vi "Calibrate DataQ.vi"() -> ()   [LabVIEW 2024]
doc: "This example performs writes and reads on a serial port, as directed by the user. You can press the Write and Read buttons, and change the Read Count, while the example is running.\n\nThe parameters set for the serial port must match the parameters of the connected instrument or device. In this example, the Read Count parameter specifies the number of bytes that the serial port reads. If there were more bytes at the port than the specified number, those bytes would not be read. If there were less bytes at the port than the specified number, you would receive a timeout error.\n\nThis example expands upon the flow control options for XON and XOFF, allowing the user to choose those control characters. Also, the user can enable or disable a termination character. Some devices require a termination character in order to identify the end of command strings. Some devices send a termination character to signify the end of data to be read. This example shows how you can end the Read operation once a termination character is detected in the buffer and/or append a termination character at the end of the Write data."
uses:
  <vilib>/Instr/_visa.llb/VISA Configure Serial Port (Instr).vi
panel:
  out "read buffer":string
  out "size(s)":i32
  in  "Correction":dbl(slide) scale=-10.0..10.0
  in  "index (row)":i32
  in  "Cal Array":dbl[][](array[numeric])
  out "Scaled":dbl
  out "Measured IN":dbl
  out "Waveform Chart":dbl[](graph)
  in  "Command List":string="stop\nencode 0\nslist 0 0\nsrate 6000\nps 2\ndec 1\ndeca 3\nnop\n\n\n"
  in  "Stop":bool
  in  "2108 CDC Virtual COM":refnum<visa-resource-name>="COM3"
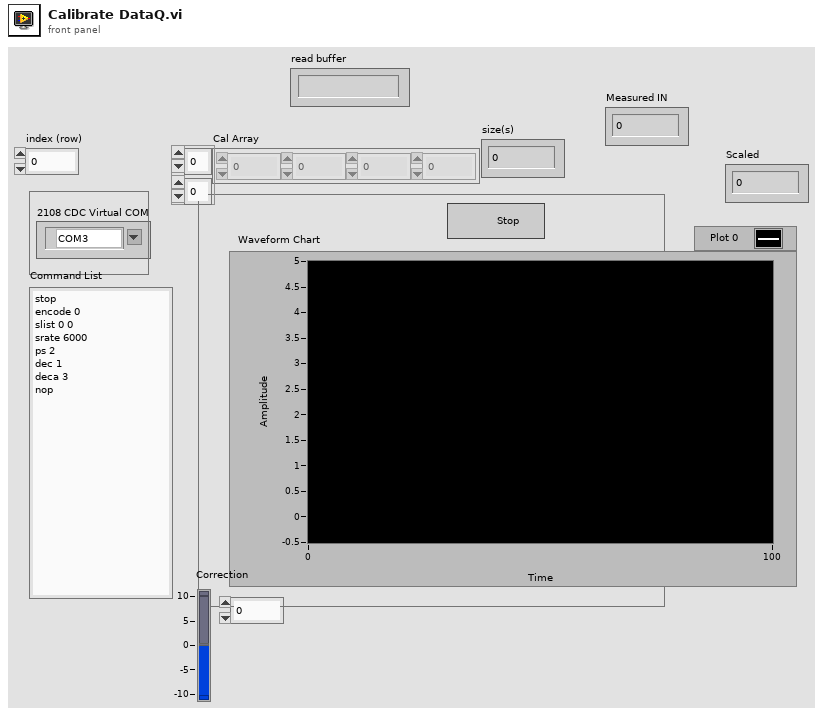
[diagram p1: front panel]
types:
  T1 = enum16{"big-endian, network order", "native, host order", "little-endian"}
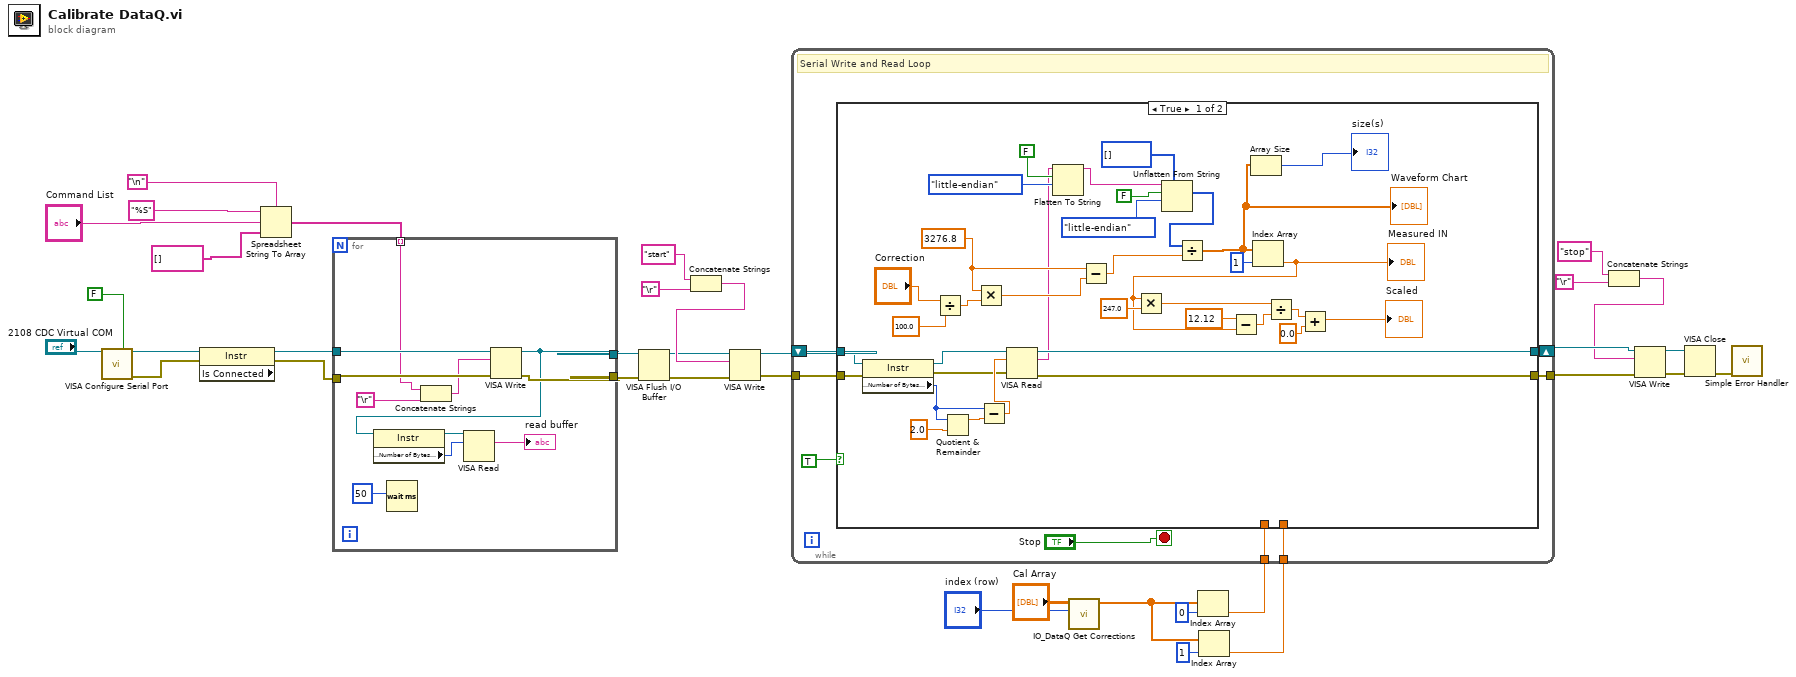
[diagram p0: block diagram]
diagram:
  n1 = call-poly "VISA Configure Serial Port"("VISA resource name"="2108 CDC Virtual COM", "Enable Termination\nChar (T)"=FALSE) -> ("VISA resource name out"=w33:refnum<visa-resource-name>, "error out"=w35:errorcluster)  [unwired: 8 in, 4 out]
  n2 = property class="Instr" props=["Is Connected"](reference=w33, error in=w35) -> (reference out=w9:refnum<visa-resource-name>, error out=w8:errorcluster)  [unwired: 1 out]
  n3 = Spreadsheet String To Array(delimiter (Tab)="\n", format string="%S", spreadsheet string="Command List", array type (2D Dbl)=string[] []) -> (array=w29:string[])
  n4 = for {
    tunnel: w29 -> [w43] mode=indexing
    tunnel: w9 -> [w46]
    tunnel: w8 -> [w45]
    tunnel: [w39] -> w13
    tunnel: [w40] -> w11
    n5 = Wait (ms)(milliseconds to wait=u32 50) -> ()  [unwired: 1 out]
    n6 = Concatenate Strings(w43, "\r") -> (w41:string)
    n7 = VISA Write(VISA resource name=w46, write buffer=w41, error in (no error)=w45) -> (VISA resource name out=w39:refnum<visa-resource-name>, error out=w40:errorcluster)  [unwired: 1 out]
    n8 = property class="Instr"(reference=w39) -> (reference out=w38:refnum<visa-resource-name>, "Serial Settings:Number of Bytes at Serial Port"=w37:u32)  [unwired: 1 in, 1 out]
    n9 = VISA Read(VISA resource name=w38, byte count=w37) -> (read buffer=→"read buffer":string)  [unwired: 1 in, 3 out]
  }
  n10 = VISA Flush I/O Buffer(VISA resource name=w13, error in (no error)=w11) -> (VISA resource name out=w12:refnum<visa-resource-name>, error out=w10:errorcluster)  [unwired: 1 in]
  n11 = Concatenate Strings("start", "\r") -> (w17:string)
  n12 = VISA Write(VISA resource name=w12, write buffer=w17, error in (no error)=w10) -> (VISA resource name out=w16:refnum<visa-resource-name>, error out=w15:errorcluster)  [unwired: 1 out]
  n13 = call "IO_DataQ Get Corrections.vi"("index (row)"="index (row)", "Cal Array"="Cal Array") -> ("Array"=w3:dbl[])  [unwired: 9 in]
  n14 = Index Array(array=w3, index=0) -> (element=w2:dbl)
  n15 = Index Array(array=w3, index=1) -> (element=w1:dbl)
  n16 = while {
    shift-right: [w54] -> w26
    shift-left: w16 -> [w51]
    tunnel: w15 -> [w50]
    tunnel: [w53] -> w23
    tunnel: w2 -> [w48]
    tunnel: w1 -> [w47]
    stop <- "Stop" stop-if-true
    # "Serial Write and Read Loop"
    n17 = case shown="True" TRUE {
      tunnel: [w89 w91] -> w54
      tunnel: w51 -> [w88 w91]
      tunnel: w50 -> [w59 w90]
      tunnel: [w83 w90] -> w53
      tunnel: w48 -> [_ _]
      tunnel: w47 -> [_ _]
      frame True {
        w62 = 3276.8
        n18 = property class="Instr"(reference=w88, error in=w59) -> (reference out=w82:refnum<visa-resource-name>, error out=w58:errorcluster, "Serial Settings:Number of Bytes at Serial Port"=w87:u32)
        n19 = Divide(x="Correction", y=100.0) -> (x/y=w63:dbl)
        n20 = Quotient & Remainder(x=w87, y=2.0) -> (x-y*floor(x/y)=w85:dbl)  [unwired: 1 out]
        n21 = Multiply(x=w62, y=w63) -> (x*y=w61:dbl)
        n22 = Subtract(x=w87, y=w85) -> (x-y=w84:dbl)
        n23 = VISA Read(VISA resource name=w82, byte count=w84, error in (no error)=w58) -> (VISA resource name out=w89:refnum<visa-resource-name>, read buffer=w57:string, error out=w83:errorcluster)  [unwired: 1 out]
        n24 = Flatten To String(anything=w57, prepend array or string size? (T)=FALSE, byte order (0:big-endian, network order)=T1."little-endian") -> (data string=w77:string)  [unwired: 1 in, 2 out]
        n25 = Subtract(x=w62, y=w61) -> (x-y=w66:dbl)
        n26 = Unflatten From String(type=i16[] [], binary string=w77, data includes array or string size? (T)=FALSE, byte order (0:big-endian, network order)=T1."little-endian") -> (value=w76:i16[])  [unwired: 1 in, 2 out]
        n27 = Divide(x=w76, y=w66) -> (x/y=w56:dbl[])
        "Waveform Chart" <- w56
        n28 = Array Size(array=w56) -> (size(s)=→"size(s)":i32)
        n29 = Index Array(array=w56, index=1) -> (element=w60:dbl)
        "Measured IN" <- w60
        n30 = Multiply(x=w60, y=247.0 ("x")) -> (x*y=w67:dbl)
        n31 = Subtract(x=12.12, y=w60) -> (x-y=w68:dbl)
        n32 = Divide(x=w67, y=w68) -> (x/y=w72:dbl)
        n33 = Add(x=w72, y=0.0) -> (x+y=→"Scaled":dbl)
      }
      frame False {
      }
    }
  }
  n34 = Concatenate Strings("stop", "\r") -> (w20:string)
  n35 = VISA Write(VISA resource name=w26, write buffer=w20, error in (no error)=w23) -> (VISA resource name out=w25:refnum<visa-resource-name>, error out=w24:errorcluster)  [unwired: 1 out]
  n36 = VISA Close(VISA resource name=w25, error in (no error)=w24) -> (error out=w34:errorcluster)
  n37 = call <vilib>:"Simple Error Handler.vi"("error in (no error)"=w34) -> ()  [unwired: 1 in, 8 out]
